vi "Extra_Gas_desk_Columns.vi"(4 "Channel Values In":string[][](array[string]), 5 "Ch names In":string[](array[string])) -> (1 "Extra Values Out":string[](array[string]), 2 "Extra Channels Out":string[](array[string]))   [LabVIEW 2010]
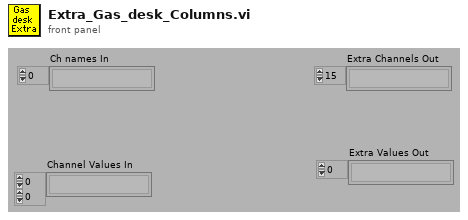
[diagram p1: front panel]
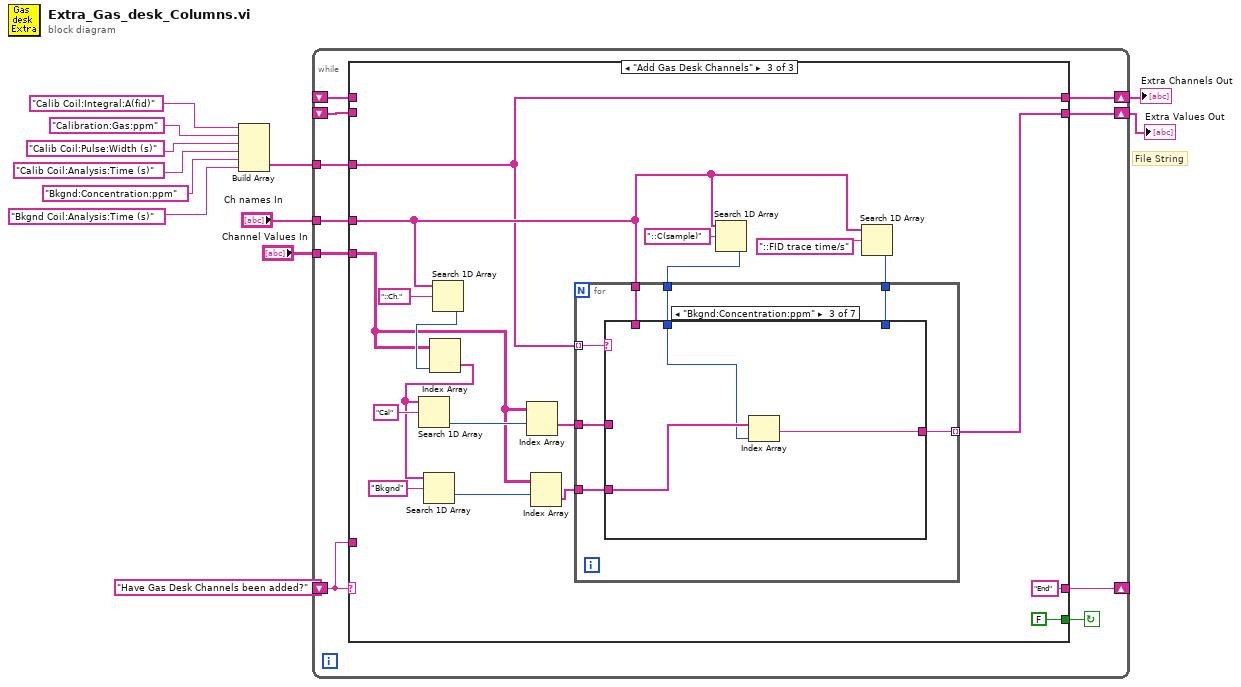
[diagram p0: block diagram]
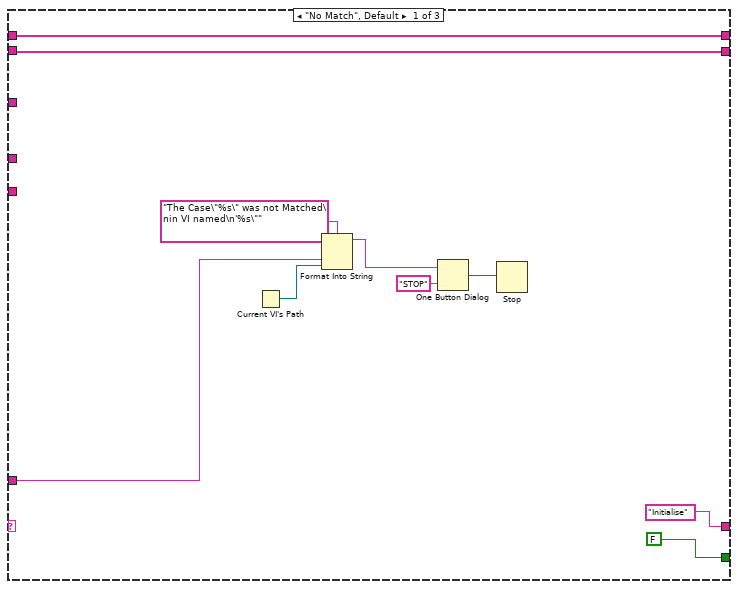
[diagram p2: hidden frame]
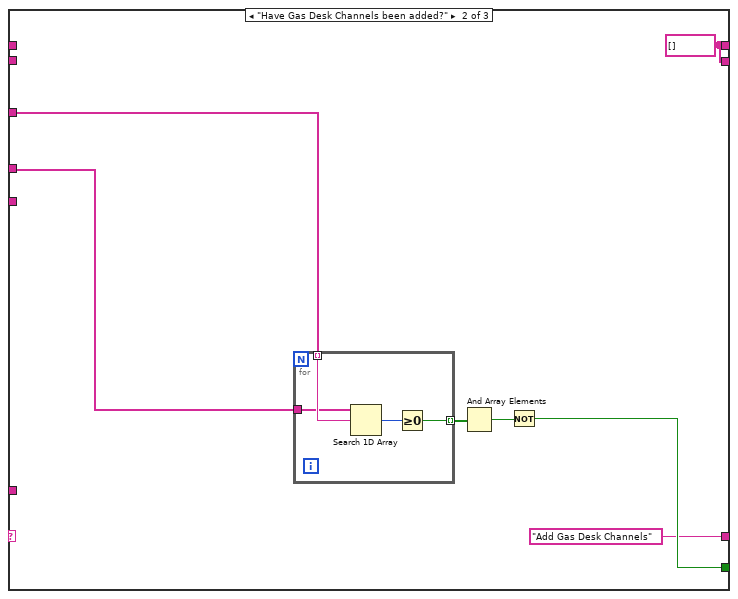
[diagram p3: hidden frame]
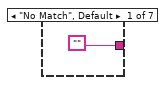
[diagram p4: hidden frame]
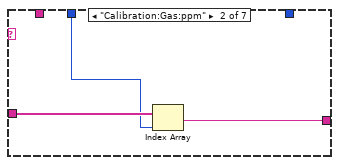
[diagram p5: hidden frame]
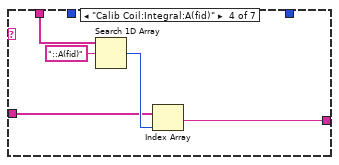
[diagram p6: hidden frame]
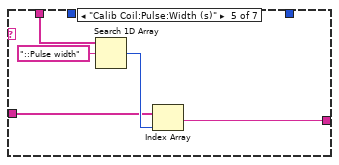
[diagram p7: hidden frame]
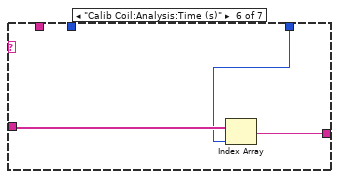
[diagram p8: hidden frame]
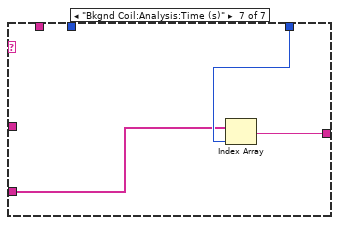
[diagram p9: hidden frame]
diagram:
  # "File String"
  n1 = Build Array("Calib Coil:Integral:A(fid)", "Calibration:Gas:ppm", "Calib Coil:Pulse:Width (s)", "Calib Coil:Analysis:Time (s)", "Bkgnd:Concentration:ppm", "Bkgnd Coil:Analysis:Time (s)") -> (w1:string[])
  n2 = while {
    tunnel: "Ch names In" -> [w15]
    tunnel: "Channel Values In" -> [w16]
    tunnel: w1 -> [w17]
    shift-left: _ -> [w18]
    shift-right: [w14] -> w8
    shift-left: _ -> [w19]
    shift-right: [w13] -> w9
    shift-left: "Have Gas Desk Channels been added?" -> [w20]
    shift-right: [w21] -> _
    stop <- w22 continue-if-true
    n3 = case shown="\"Add Gas Desk Channels\"" w20 {
      tunnel: [FALSE w34 FALSE] -> w22
      tunnel: ["Initialise" "Add Gas Desk Channels" "End" ("f")] -> w21
      tunnel: w20 -> [w27 _ _]
      tunnel: w19 -> [w24 _ _]
      tunnel: w18 -> [w23 _ _]
      tunnel: w17 -> [_ w38 w45]
      tunnel: w16 -> [_ _ w47]
      tunnel: w15 -> [_ w37 w46]
      tunnel: [w24 w36 w45] -> w13
      tunnel: [w23 w36 w44] -> w14
      frame "No Match", Default {
        n4 = Current VI's Path() -> (path=w26:path)
        n5 = Format Into String(format string="The Case\"%s\" was not Matched\nin VI named\n'%s\"" ("Format String"), w27, w26) -> (resulting string=w30:string)  [unwired: 2 in, 1 out]
        n6 = One Button Dialog(message=w30, button name ("OK")="STOP") -> (true=w28:bool)
        n7 = Stop(stop? (T)=w28) -> ()
      }
      frame "Have Gas Desk Channels been added?" {
        w36 = string[] []
        n8 = for {
          tunnel: w38 -> [w41] mode=indexing
          tunnel: [w42] -> w39 mode=indexing
          tunnel: w37 -> [w40]
          n9 = Search 1D Array(1D array=w40, element=w41) -> (index of element=w43:i32)  [unwired: 1 in]
          n10 = Greater Or Equal To 0?(x=w43) -> (x >= 0?=w42:bool)
        }
        n11 = And Array Elements(Boolean array=w39) -> (logical AND=w35:bool)
        n12 = Not(x=w35) -> (.not. x?=w34:bool)
      }
      frame "Add Gas Desk Channels" {
        n13 = Search 1D Array(1D array=w46, element="::Ch.") -> (index of element=w58:i32)  [unwired: 1 in]
        n14 = Index Array(array=w47, index (col)=w58) -> (element=w57:string[])  [unwired: 1 in]
        n15 = Search 1D Array(1D array=w57, element="Cal") -> (index of element=w55:i32)  [unwired: 1 in]
        n16 = Search 1D Array(1D array=w57, element="Bkgnd") -> (index of element=w56:i32)  [unwired: 1 in]
        n17 = Index Array(array=w47, index (row)=w55) -> (element=w54:string[])  [unwired: 1 in]
        n18 = Index Array(array=w47, index (row)=w56) -> (element=w53:string[])  [unwired: 1 in]
        n19 = Search 1D Array(1D array=w46, element="::C(sample)") -> (index of element=w50:i32)  [unwired: 1 in]
        n20 = Search 1D Array(1D array=w46, element="::FID trace time/s") -> (index of element=w49:i32)  [unwired: 1 in]
        n21 = for {
          tunnel: w45 -> [w69] mode=indexing
          tunnel: w46 -> [w68]
          tunnel: w54 -> [w67]
          tunnel: [w66] -> w44 mode=indexing
          tunnel: w53 -> [w65]
          tunnel: w50 -> [w64]
          tunnel: w49 -> [w63]
          n22 = case shown="\"Bkgnd:Concentration:ppm\"" w69 {
            tunnel: w68 -> [_ _ _ w81 w86 _ _]
            tunnel: w67 -> [_ w73 _ w77 w82 w88 _]
            tunnel: ["" w72 w76 w78 w83 w89 w92] -> w66
            tunnel: w65 -> [_ _ w75 _ _ _ w90]
            tunnel: w64 -> [_ w71 w74 _ _ _ _]
            tunnel: w63 -> [_ _ _ _ _ w87 w91]
            frame "No Match", Default {
            }
            frame "Calibration:Gas:ppm" {
              n23 = Index Array(array=w73, index=w71) -> (element=w72:string)
            }
            frame "Bkgnd:Concentration:ppm" {
              n24 = Index Array(array=w75, index=w74) -> (element=w76:string)
            }
            frame "Calib Coil:Integral:A(fid)" {
              n25 = Search 1D Array(1D array=w81, element="::A(fid)") -> (index of element=w79:i32)  [unwired: 1 in]
              n26 = Index Array(array=w77, index=w79) -> (element=w78:string)
            }
            frame "Calib Coil:Pulse:Width (s)" {
              n27 = Search 1D Array(1D array=w86, element="::Pulse width") -> (index of element=w84:i32)  [unwired: 1 in]
              n28 = Index Array(array=w82, index=w84) -> (element=w83:string)
            }
            frame "Calib Coil:Analysis:Time (s)" {
              n29 = Index Array(array=w88, index=w87) -> (element=w89:string)
            }
            frame "Bkgnd Coil:Analysis:Time (s)" {
              n30 = Index Array(array=w90, index=w91) -> (element=w92:string)
            }
          }
        }
      }
    }
  }
  "Extra Channels Out" <- w9
  "Extra Values Out" <- w8
